vi "RML Parsing.vi"(8 "error in (no error)":errorcluster, 10 "XML String":string="<?xml version=\"1.0\" encoding=\"ISO-8859-1\"?>\n<bookstore>\n<book ISBN=\"978-0545128285\">\n  <title lang=\"en\">The Tales of Beedle the Bard</title>\n  <author>J. K. Rowling</author>\n  <year>2008</year>\n  <price>12.99</price>\n</book>\n<book ISBN=\"978-0316160209\">\n  <title lang=\"en\">Eclipse</title>\n  <author>Stephenie Meyer</author>\n  <year>2007</year>\n  <price>19.99</price>\n</book>\n<book ISBN=\"978-0316067928\">\n  <title lang=\"en\">Breaking Dawn</title>\n  <author>Stephenie Meyer</author>\n  <year>2008</year>\n  <price>22.99</price>\n</book>\n<book ISBN=\"978-0316017923\">\n  <title lang=\"en\">Outliers: The Story of Success</title>\n  <author>Malcolm Gladwell</author>\n  <year>2008</year>\n  <price>27.99</price>\n</book>\n<book ISBN=\"978-0596007645\">\n  <title lang=\"en\">XML in a Nutshell</title>\n  <author>Elliotte Rusty Harold</author>\n  <author>W. Scott Means</author>\n  <year>2004</year>\n  <price>39.95</price>\n</book>\n</bookstore>", 11 "XPath Expression":string="/bookstore/book/title") -> (0 "error out":errorcluster, 3 "Search Results":string[](array[string]))   [LabVIEW 2018]
doc: "This example demonstrates how to query an XML document by using an XPath expression and returns all the nodes that match the XPath expression."
uses:
  <vilib>/xml/Load XML String.vi
  <vilib>/xml/Close Reference(Node).vi
  <resource>/objmgr/DOMUserDefRef.rc
  <vilib>/xml/NI_XML.lvlib
panel:
  # "Overview: Demonstrates the use of the XML Parser VIs and functions to search an XML string for multiple nodes (tags) that match a given XPath search expression.\nInstructions:\nRun the VI."
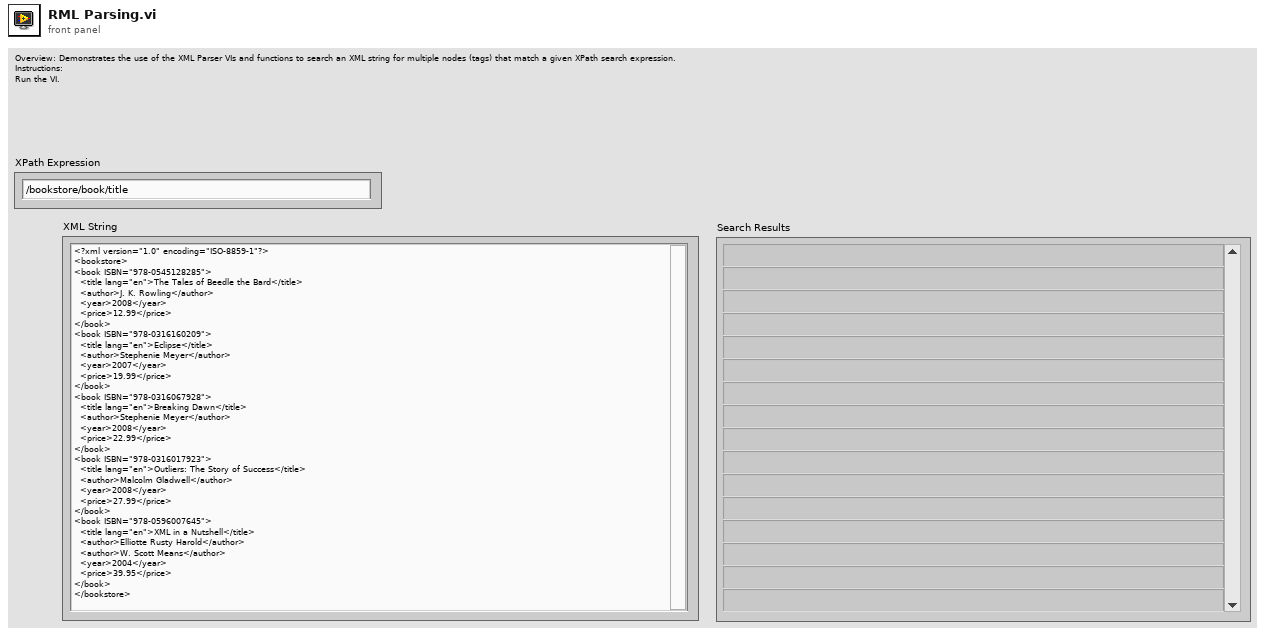
[diagram p1: front panel]
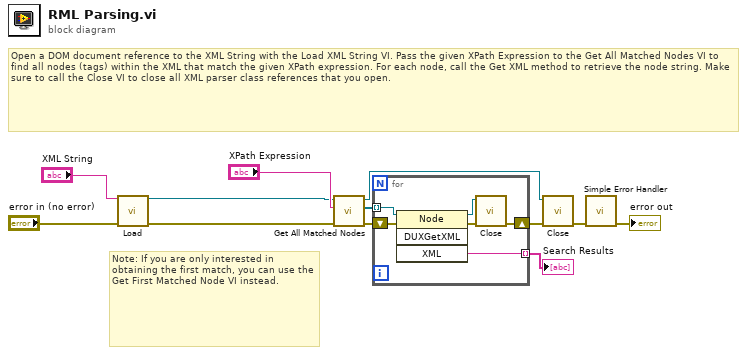
[diagram p0: block diagram]
diagram:
  # "Note: If you are only interested in obtaining the first match, you can use the Get First Matched Node VI instead."
  # "Open a DOM document reference to the XML String with the Load XML String VI. Pass the given XPath Expression to the Get All Matched Nodes VI to find all nodes (tags) within the XML that match the given XPath expression. For each node, call the Get XML method to retrieve the node string. Make sure to call the Close VI to close all XML parser class references that you open."
  n1 = call-poly <vilib>:"Load.vi"("XML string"="XML String", "error in (no error)"="error in (no error)") -> ("DOM document out"=w4:refnum<k20>, "error out"=w3:errorcluster)  [unwired: 11 in, 1 out]
  n2 = call <vilib>:"Get All Matched Nodes.vi"("error in (no error)"=w3, "XPath expression"="XPath Expression", "node in"=w4) -> ("error out"=w11:errorcluster, "node result array"=w12:refnum<k20>[], "node out"=w8:refnum<k20>)  [unwired: 6 out]
  n3 = for {
    tunnel: w12 -> [w14] mode=indexing
    shift-right: [w16] -> w9
    shift-left: w11 -> [w15]
    tunnel: [w13] -> w6 mode=indexing
    n4 = invoke on="Invoke Node" class="Node" method="DUXGetXML"(reference=w14, error in=w15) -> (reference out=w17:refnum<k20>, error out=w18:errorcluster, "XML"=w13:string)  [unwired: 2 in, 1 out]
    n5 = call-poly <vilib>:"Close.vi"("error in (no error)"=w18, "node"=w17) -> ("error out"=w16:errorcluster)  [unwired: 7 out]
  }
  "Search Results" <- w6
  n6 = call-poly <vilib>:"Close.vi"("error in (no error)"=w9, "node"=w8) -> ("error out"=w7:errorcluster)  [unwired: 7 out]
  n7 = call <vilib>:"Simple Error Handler.vi"("error in (no error)"=w7) -> ("error out"=→"error out":errorcluster)  [unwired: 1 in, 7 out]
